vi "Colors.vi"(2 "Pixels colors (uchar)":u32[](array[numeric]), 3 "stdout":string, 7 "TracesRead error":errorcluster) -> (11 "Colors error":errorcluster, 13 "Number of Traces":i32, 14 "Corners color (CLUT)":i32, 15 "Corners":u32(colorbox), 16 "Traces":u32[](array[colorbox]), 17 "Traces colors string (RGB)":string[](array[string]), 18 "Traces colors (CLUT)":i32[](array[numeric]), 19 "Traces colors (RGB)":u8[][](array[numeric]))   [LabVIEW 2023]
uses:
  <vilib>/Utility/error.llb/Trim Whitespace One-Sided.vi
panel:
  in  "User interface":T1(tab)
  in  "User entries":enum32{""}(tab)
  in  "Customization":enum32{"Customization"}(tab)
  in  "Colors":enum32{"Colors"}(tab)
  in  "Size":enum32{"Size"}(tab)
  in  "Loop FOR 1":enum32{"Loop FOR 1"}(tab)
  out "appended array":u8[](array[numeric])
  out "Color CLUT at index I":u32
  out "Color Box":u32(colorbox)
  out "B":u8
  out "G":u8
  out "R":u8
  in  "Arrays":enum32{"Arrays"}(tab)
  in  "Script.m":enum32{"Script.m"}(tab)
  in  "Extract.c output string scan":enum32{"Extract.c output string scan"}(tab)
  in  "T: tt1 tt2 tt3 ...":enum32{"T: tt1 tt2 tt3 ..."}(tab)
  out "before substring \"T:\"":string
  out "after substring \"T:\"":string
  in  "C: cc":enum32{"C: cc"}(tab)
  out "string out":string
  in  "Loop FOR 2":enum32{"Loop FOR 2"}(tab)
  out "Array RGB to Array string":string
  in  "LabVIEW":enum32{"LabVIEW"}(tab)
  in  "MATLAB":enum32{"MATLAB"}(tab)
  in  "C":enum32{"C"}(tab)
  in  "MATLAB":enum32{"MATLAB"}(tab)
  in  "C":enum32{"C"}(tab)
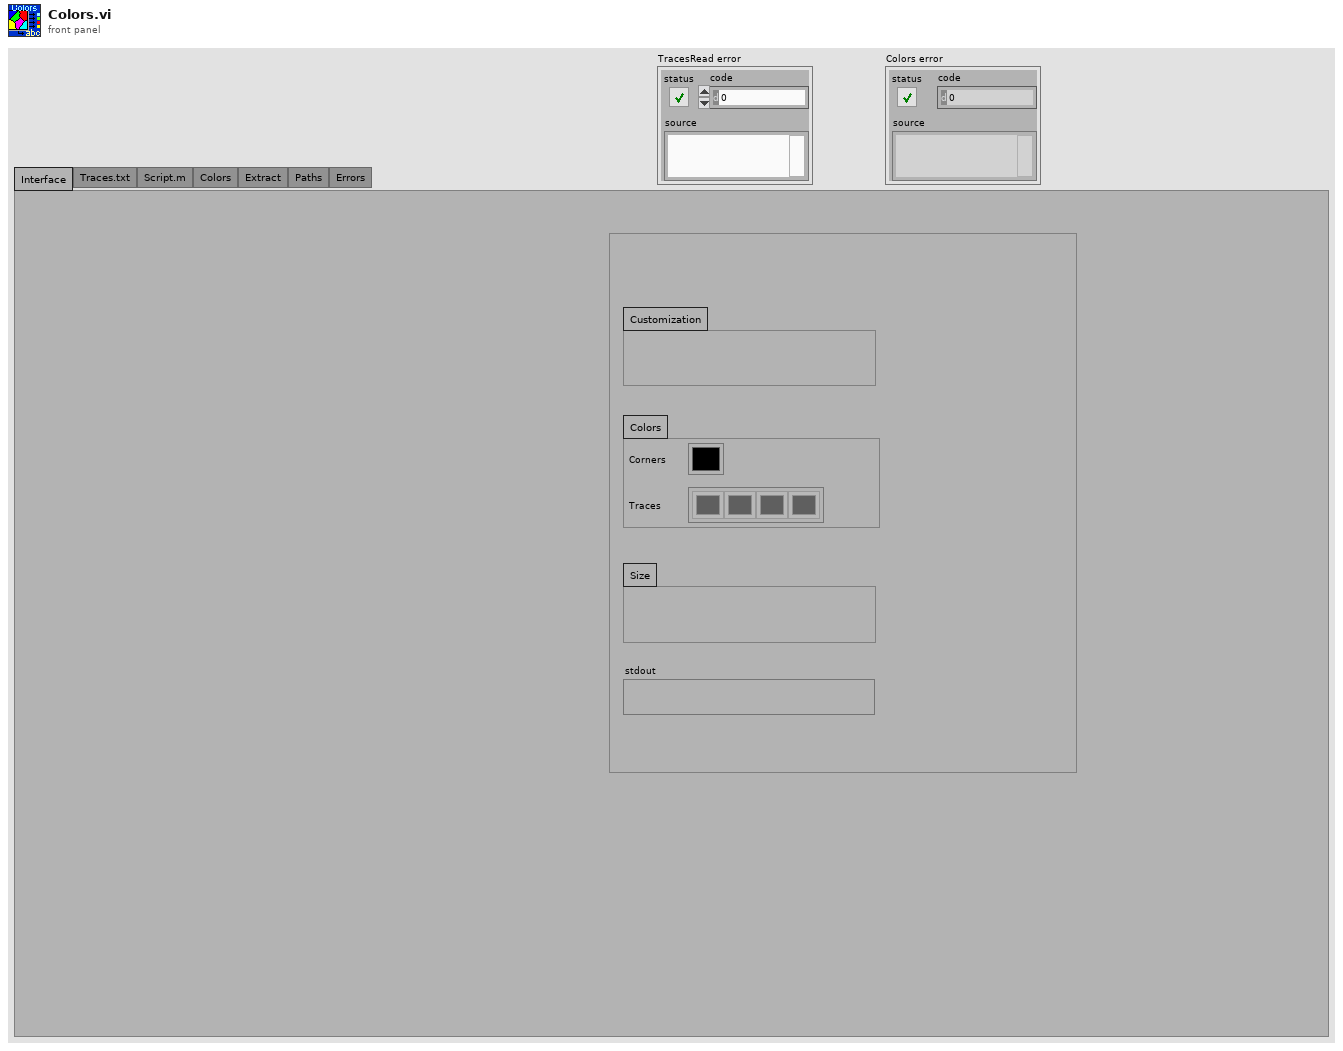
[diagram p1: front panel]
types:
  T1 = enum32{"Interface", "Traces.txt", "Script.m", "Colors", "Extract", "Paths", "Errors"}
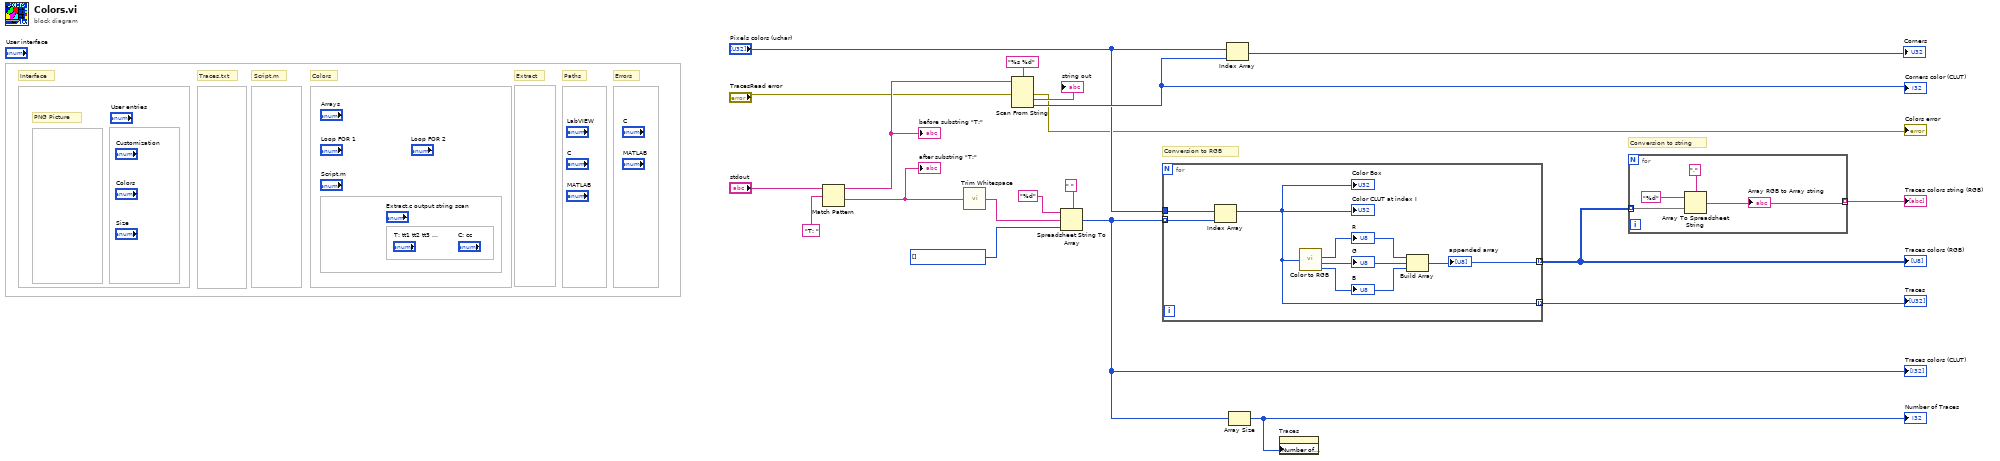
[diagram p0: block diagram]
diagram:
  # "Conversion to RGB"
  # "Conversion to string"
  # "PNG Picture"
  # "Errors"
  # "Paths"
  # "Extract"
  # "Colors"
  # "Script.m"
  # "Traces.txt"
  # "Interface"
  n1 = Match Pattern(string="stdout", regular expression="T: ") -> (before substring=w15:string, after substring=w12:string)  [unwired: 1 in, 2 out]
  "after substring \"T:\"" <- w12
  "before substring \"T:\"" <- w15
  n2 = call <vilib>:"Trim Whitespace.vi"("string"=w12) -> ("trimmed string"=w11:string)  [unwired: 1 in]
  n3 = Scan From String(format string="%s %d", input string=w15, error in="TracesRead error") -> (error out=→"Colors error":errorcluster, output 1=→"string out":string, output 2=w19:i32)  [unwired: 3 in, 2 out]
  "Corners color (CLUT)" <- w19
  n4 = Spreadsheet String To Array(delimiter (Tab)=" ", format string="%d", spreadsheet string=w11, array type (2D Dbl)=i32[] []) -> (array=w9:i32[])
  "Traces colors (CLUT)" <- w9
  n5 = for {
    tunnel: w9 -> [w27] mode=indexing
    tunnel: "Pixels colors (uchar)" -> [w26]
    tunnel: [w25] -> w10 mode=indexing
    tunnel: [w21] -> w7 mode=indexing
    n6 = Index Array(array=w26, index=w27) -> (element=w25:u32)
    "Color CLUT at index I" <- w25
    "Color Box" <- w25
    n7 = call <vilib>:"Color to RGB.vi"("Color"=w25) -> ("R"=w24:u8, "G"=w23:u8, "B"=w22:u8)  [unwired: 1 out]
    "R" <- w24
    "G" <- w23
    "B" <- w22
    n8 = Build Array(w24, w23, w22) -> (w21:u8[])
    "appended array" <- w21
  }
  "Traces" <- w10
  "Traces colors (RGB)" <- w7
  n9 = Index Array(array="Pixels colors (uchar)", index=w19) -> (element=→"Corners":u32)
  n10 = Array Size(array=w9) -> (size(s)=w8:i32)
  "Number of Traces" <- w8
  n11 = property on="Traces" class="Arr (strict)"("Number of Columns"=w8) -> ()  [unwired: 2 in, 2 out]
  n12 = for {
    tunnel: w7 -> [w31] mode=indexing
    tunnel: [w28] -> w6 mode=indexing
    n13 = Array To Spreadsheet String(delimiter (Tab)=",", array=w31, 3:"%d" ("format string")) -> (spreadsheet string=w28:string)
    "Array RGB to Array string" <- w28
  }
  "Traces colors string (RGB)" <- w6
